vi "field setpoint4(SubVI).vi"(0 "Filed 2":dbl=300.0, 1 "Field":dbl=300.0, 3 "Rate":dbl=10.0, 4 "Mode":i32(ring) items=["Persistent", "Driven"], 5 "Instrument Ref":refnum<k24>, 6 "data":refnum<queue>, 7 "Delay":dbl, 9 "steps number":i32, 11 "Approach":i32(ring) items=["FastSettle", "NoOvershoot"], 12 "ch str":string, 13 "Resource In":refnum<visa-resource-name>, 15 "abort":refnum<queue>) -> (8 "错误输出":errorcluster)   [LabVIEW 2019, in "SubVI.lvlib"]
uses:
  SubVI.lvlib
  C:/Users/jigui/Desktop/6021c3341675da1470d48a46f17edaef7a5b42f5/QDInstrument_LabView (1)/QDInstrument.dll
  QDInstrument_LabView (1)/QDInstrument.dll
panel:
  out "数组":dbl[](array[numeric])
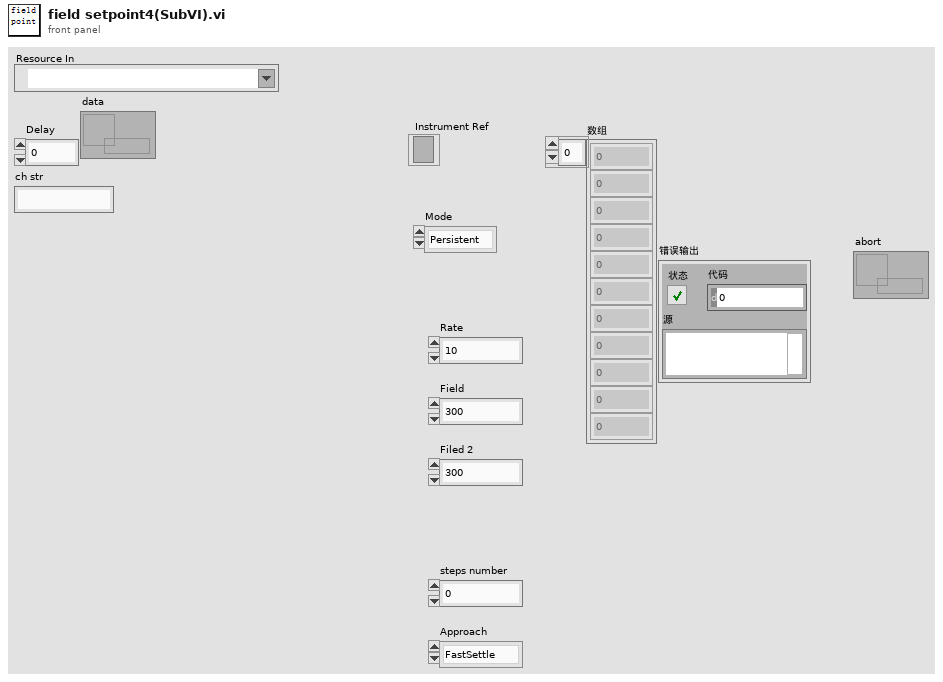
[diagram p1: front panel]
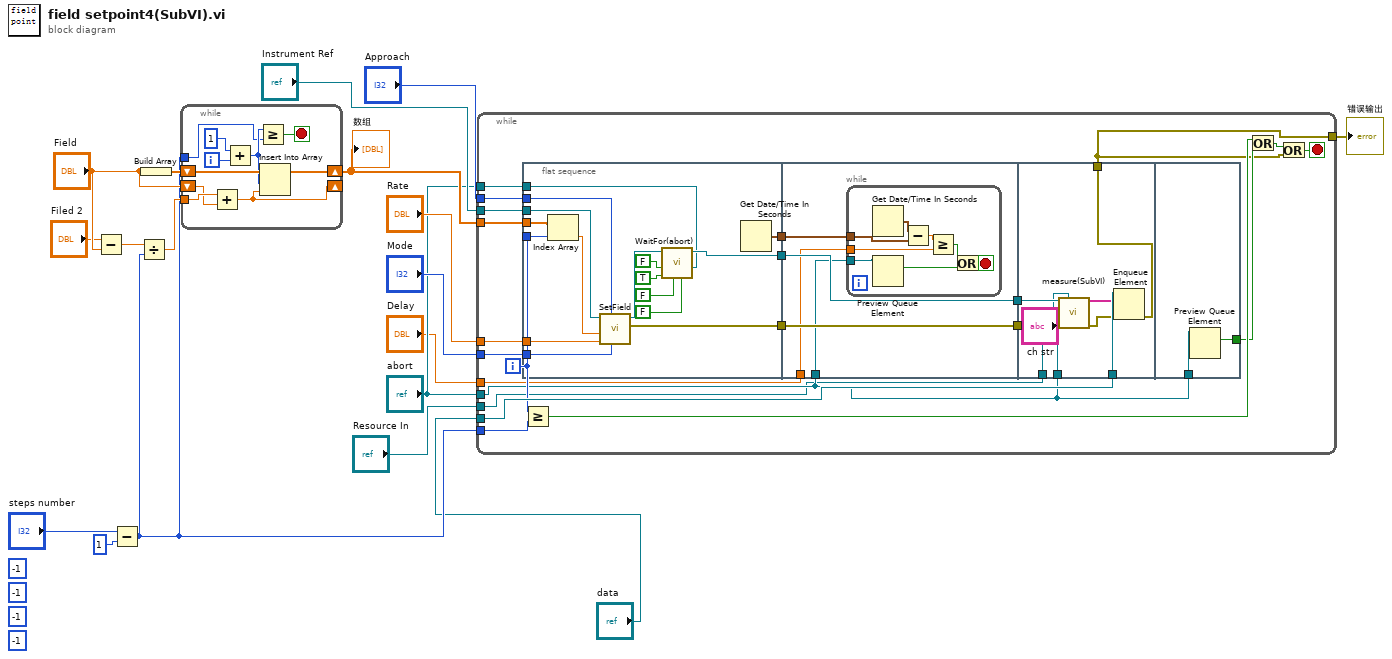
[diagram p0: block diagram]
diagram:
  (unwired) -1 ("量程结束")
  (unwired) -1 ("量程结束")
  (unwired) -1 ("量程结束")
  (unwired) -1 ("量程结束")
  n1 = Subtract(x="Filed 2", y="Field") -> (x-y=w15:dbl)
  n2 = Subtract(x="steps number", y=1) -> (x-y=w4:i32)
  n3 = Divide(x=w15, y=w4) -> (x/y=w17:dbl)
  n4 = Build Array("Field") -> (w16:dbl[])
  n5 = while {
    shift-right: [w28] -> w10
    shift-left: w16 -> [w27]
    tunnel: w17 -> [w22]
    tunnel: w4 -> [w21]
    shift-right: [w20] -> _
    shift-left: "Field" -> [w19]
    i -> [w26]
    stop <- w23 stop-if-true
    n6 = Add(x=w22, y=w19) -> (x+y=w20:dbl)
    n7 = Add(x=1, y=w26) -> (x+y=w24:i32)
    n8 = Greater Or Equal?(x=w24, y=w21) -> (x >= y?=w23:bool)
    n9 = Insert Into Array(array=w27, index=w24, new element=w20) -> (w28:dbl[])
  }
  "数组" <- w10
  n10 = while {
    tunnel: w4 -> [w47]
    tunnel: "data" -> [w50]
    tunnel: "abort" -> [w30]
    tunnel: "Mode" -> [w45]
    tunnel: "Approach" -> [w44]
    tunnel: "Rate" -> [w43]
    tunnel: "Instrument Ref" -> [w42]
    tunnel: w10 -> [w41]
    tunnel: "abort" -> [w40]
    tunnel: [w37] -> w7
    tunnel: "Delay" -> [w31]
    tunnel: "Resource In" -> [w29]
    i -> [w46]
    stop <- w38 stop-if-true
    n11 = flat-sequence {
      tunnel: [w58] -> w36
      tunnel: w46 -> [w61]
      tunnel: w45 -> [w65]
      tunnel: w44 -> [w64]
      tunnel: w43 -> [w63]
      tunnel: w42 -> [w60]
      tunnel: w41 -> [w62]
      tunnel: w40 -> [w53]
      tunnel: [w52] -> w34
      tunnel: [w51] -> w32
      tunnel: w36 -> [w71]
      tunnel: [w71] -> w35
      tunnel: w34 -> [w70]
      tunnel: [w70] -> w33
      tunnel: w32 -> [w69]
      tunnel: w31 -> [w68]
      tunnel: w30 -> [w67]
      tunnel: w35 -> [w88]
      tunnel: w50 -> [w87]
      tunnel: w30 -> [w83]
      tunnel: w33 -> [w85]
      tunnel: [w81] -> w37
      tunnel: w29 -> [w84]
      tunnel: w30 -> [w90]
      tunnel: [w89] -> w48
      frame #0 {
        n12 = Index Array(array=w62, index=w61) -> (element=w66:dbl)
        n13 = call "SetField.vi"("Mode"=w65, "Approach"=w64, "Rate"=w63, "Field"=w66, "Instrument Ref In"=w60) -> ("error out"=w52:errorcluster, "Instrument Ref Out"=w59:refnum<k24>)  [unwired: 2 in, 1 out]
        n14 = call "WaitFor(abort).vi"("abort"=w53, "Wait For Chamber"=FALSE, "Wait For Position"=FALSE, "Wait For Field"=TRUE, "Wait For Temperature"=FALSE, "Instrument Ref In"=w59) -> ("Instrument Ref Out"=w58:refnum<k24>)  [unwired: 4 in, 1 out]
        n15 = Get Date/Time In Seconds() -> (seconds since 1Jan1904=w51:timestamp)
      }
      frame #1 {
        n16 = while {
          tunnel: w69 -> [w78]
          tunnel: w68 -> [w76]
          tunnel: w67 -> [w74]
          stop <- w72 stop-if-true
          n17 = Get Date/Time In Seconds() -> (seconds since 1Jan1904=w79:timestamp)
          n18 = Preview Queue Element(queue=w74) -> (element=w73:bool)  [unwired: 2 in, 3 out]
          n19 = Subtract(x=w79, y=w78) -> (x-y=w77:dbl)
          n20 = Greater Or Equal?(x=w77, y=w76) -> (x >= y?=w75:bool)
          n21 = Or(x=w75, y=w73) -> (x .or. y?=w72:bool)
        }
      }
      frame #2 {
        n22 = call "measure(SubVI).vi"(".NET引用句柄输入"=w88, "error"=w83, "Resource In"=w84, "error in (no error)"=w85, "ch str"="ch str") -> ("data"=w86:string[], "error out"=w82:errorcluster)  [unwired: 9 in]
        n23 = Enqueue Element(queue=w87, element=w86, error in (no error)=w82) -> (error out=w81:errorcluster)  [unwired: 1 in, 2 out]
      }
      frame #3 {
        n24 = Preview Queue Element(queue=w90) -> (element=w89:bool)  [unwired: 2 in, 3 out]
      }
    }
    n25 = Greater Or Equal?(x=w46, y=w47) -> (x >= y?=w49:bool)
    n26 = Or(x=w49, y=w48) -> (x .or. y?=w39:bool)
    n27 = Or(x=w39, y=w37) -> (x .or. y?=w38:bool)
  }
  "错误输出" <- w7
